vi "Write Horizontal Scrollbar.vi"(10 "Horizontal Scrollbar":bool, 11 "Flex Subpanel in":refnum<class "Flex UI Subpanel.lvclass">) -> (3 "Flex Subpanel out":refnum<class "Flex UI Subpanel.lvclass">)   [LabVIEW 2016, in "Flex UI Subpanel.lvclass"]
uses:
  Flex UI Subpanel.lvclass
  Flex UI Subpanel.lvclass/Flex UI Subpanel.ctl
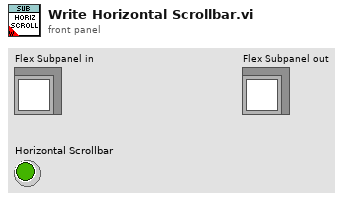
[diagram p1: front panel]
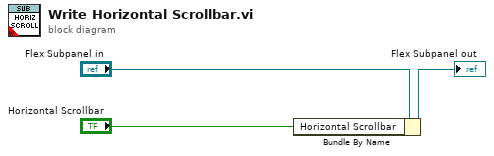
[diagram p0: block diagram]
diagram:
  n1 = Bundle By Name(cluster="Flex Subpanel in", "Horizontal Scrollbar"="Horizontal Scrollbar") -> (→"Flex Subpanel out":refnum<class "Flex UI Subpanel.lvclass">)
